vi "Get Time in Second with Error Input.vi"(3 "Error in":errorcluster caption="Error in (no error)") -> (0 "Error out":errorcluster, 1 "current time":timestamp)   [LabVIEW 2017]
doc: "Returns the current time in seconds as a timestamp and passes the error cluster through."
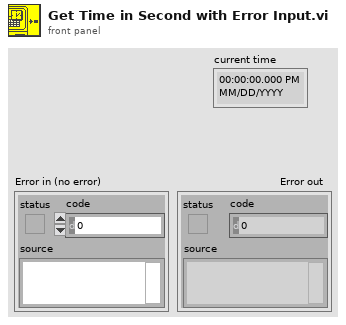
[diagram p1: front panel]
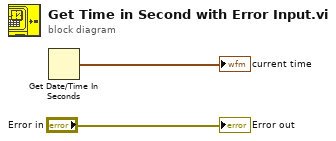
[diagram p0: block diagram]
diagram:
  n1 = Get Date/Time In Seconds() -> (seconds since 1Jan1904=→"current time":timestamp)
  "Error out" <- "Error in"
